vi "TCP IP Parse CutMode.vi"(11 "JSON in":string) -> (2 "Value":T1, 3 "JSON out":string)   [LabVIEW 2015]
uses:
  Controls/Control_Fornax Mono1 Cut Enum.ctl
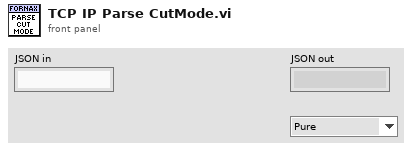
[diagram p1: front panel]
types:
  T1 = typedef "Control_Fornax Mono1 Cut Enum.ctl" = enum16{"Pure", "Blend"}
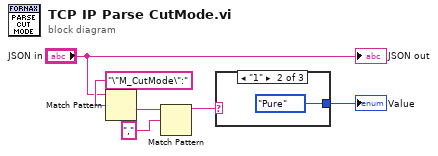
[diagram p0: block diagram]
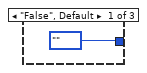
[diagram p2: hidden frame]
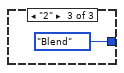
[diagram p3: hidden frame]
diagram:
  n1 = Match Pattern(string="JSON in", regular expression="\"M_CutMode\":") -> (after substring=w4:string)  [unwired: 1 in, 3 out]
  n2 = Match Pattern(string=w4, regular expression=",") -> (before substring=w6:string)  [unwired: 1 in, 3 out]
  n3 = case shown="\"1\"" w6 {
    tunnel: [enum16{""}."" Control_Fornax_Mono1_Cut_Enum."Pure" ("Value") Control_Fornax_Mono1_Cut_Enum."Blend" ("Value")] -> w1
    frame "False", Default {
    }
    frame "1" {
    }
    frame "2" {
    }
  }
  "Value" <- w1
  "JSON out" <- "JSON in"
